vi "TCP-Ping.vi"(0 "IP Address":string, 5 "Port":i32, 11 "error in (no error)":errorcluster) -> (15 "error out":errorcluster)   [LabVIEW 2020]
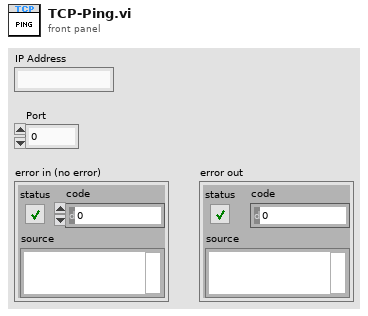
[diagram p1: front panel]
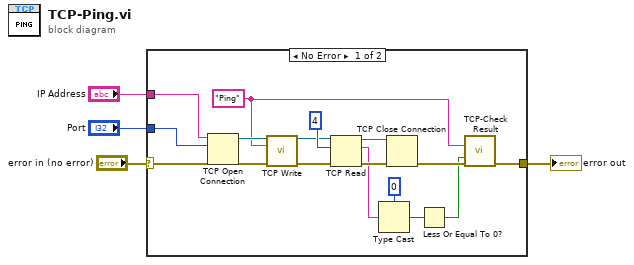
[diagram p0: block diagram]
diagram:
  n1 = case shown="No Error" "error in (no error)" {
    selector: "error in (no error)" -> [w16 w22]
    tunnel: "Port" -> [w13 _]
    tunnel: "IP Address" -> [w12 _]
    tunnel: [w9 w22] -> w1
    frame No Error {
      w10 = "Ping" ("data string")
      n2 = TCP Open Connection(address=w12, remote port or service name=w13, error in (no error)=w16) -> (connection ID=w15:refnum<k5>, error out=w14:errorcluster)  [unwired: 2 in]
      n3 = call "TCP Write.vi"("connection ID"=w15, "data string"=w10, "error in (no error)"=w14) -> ("connection ID out"=w18:refnum<k5>, "error out"=w17:errorcluster)  [unwired: 10 in, 1 out]
      n4 = TCP Read(connection ID=w18, bytes to read=4, error in (no error)=w17) -> (connection ID out=w21:refnum<k5>, data out=w8:string, error out=w20:errorcluster)  [unwired: 2 in]
      n5 = Type Cast(type=0 ("bytes to read"), x=w8) -> (*(type *) &x=w6:i32)
      n6 = TCP Close Connection(connection ID=w21, error in (no error)=w20) -> (error out=w11:errorcluster)  [unwired: 1 in, 1 out]
      n7 = Less Or Equal To 0?(x=w6) -> (x <= 0?=w5:bool)
      n8 = call "TCP-Check Result.vi"("command"=w10, "invalid response"=w5, "error IO"=w11) -> ("error out"=w9:errorcluster)  [unwired: 12 in]
    }
    frame Error {
    }
  }
  "error out" <- w1
